vi "Create Default Attributes.vi"(5 "Unique ID":string, 7 "Process Executive Ref":refnum<data-value>, 11 "Start Air Dry in":refnum<class "Start Air Dry.lvclass">) -> (3 "Start Air Dry out":refnum<class "Start Air Dry.lvclass">)   [LabVIEW 2019, in "Start Air Dry.lvclass"]
uses:
  <vilib>/gpm_packages/@cs/Car-wash/Source/Process Steps/Start Air Dry/Start Air Dry.lvclass
  <vilib>/gpm_packages/@cs/test-executive/Source/Test Executive/ITestExecutive/ITest Executive.lvclass
  446e14c0-bd35-41e7-82a1-fb070b80a9cb.vi
  <vilib>/Utility/error.llb/Error Cluster From Error Code.vi
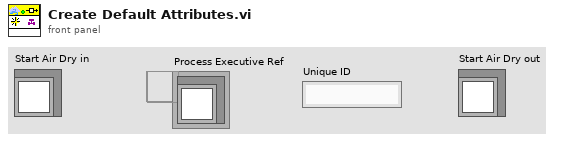
[diagram p1: front panel]
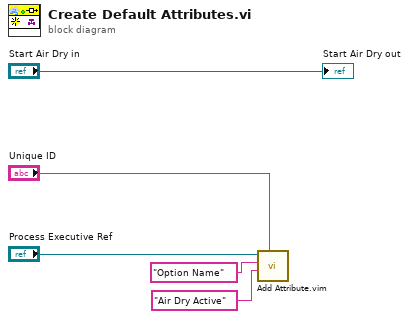
[diagram p0: block diagram]
diagram:
  n1 = call "Add Attribute.vim"("ID"="Unique ID", "Attribute"="Air Dry Active" ("Item Name"), "Attribute Name"="Option Name" ("Item Name"), "Test Executive Ref"="Process Executive Ref") -> ()  [unwired: 4 in, 4 out]
  "Start Air Dry out" <- "Start Air Dry in"
